vi "Engine-Throttle-Host.vi"() -> ()   [LabVIEW 2016]
panel:
  in  "_Hidden":enum32{"Page 1"}(tab)
  out "TB1_DisHHChans":sgl[](array[numeric])
  out "TB2_DisHHChans":sgl[](array[numeric])
  out "TB1_DC":sgl
  out "TB2_DC":sgl
  out "TB1_Polarity":bool
  out "TB2_Polarity":bool
  out "TB1_Fault":bool
  out "TB2_Fault":bool
  out "TB2_ModeStatus":T1(ring)
  in  "TB2_ModeSelect":T1(ring)
  in  "TB2_ControlEnable":bool
  in  "TB2_Psn_Req":sgl caption="TB1_PsnReq" format="%3_3g"
  out "TB2_Primary":sgl format="%3_3g"
  in  "TB1_ModeSelect":T1(ring)
  out "TB1_Primary":sgl format="%3_3g"
  in  "TB1_ControlEnable":bool
  in  "TB1_Psn_Req":sgl caption="TB1_PsnReq" format="%3_3g"
  out "TB1_ModeStatus":T1(ring)
  in  "_ThrottleTab":enum32{"Throttle 1", "Throttle 2"}(tab)
  in  "_ParameterTab":T2(tab)
  in  "TB1_CtrlCal":T3={"TLead [sec]"=0.0, "TLag [sec]"=0.1, "KRpos [V/ ]"=0.5, "TIpos [sec]"=0.15, "TDpos [sec]"=0.01, "KRneg [V/ ]"=1.0, "TIneg [sec]"=0.1, "TDneg [sec]"=0.001, "LH Position Band"=0.2, "U LH (V)"=2.0, "U LH Lag [sec]"=0.06, "US (V)"=0.5, "US Lag [sec]"=0.15, "LH Position"=5.0, "Motor Resistance"=2.4, "Position Fault Thresh"=10.0} caption="Control Calibration" {"LH Position" format="%.3f"; "U LH Lag [sec]" format="%.3f"; "US Lag [sec]" format="%.3f"; "TLead [sec]" format="%.3f"; "TLag [sec]" format="%.3f"}
  in  "TB1_PsnCalIn":T4 caption="Position Calibration In"
  in  "TB1_PsnCalSettings":T5={"Psn Cal Init Delay (sec)"=1.0, "u Psn Cal Inc (V)"=0.2, "u Psn Cal Inc Thresh (V)"=1.1, "Psn Cal Return From Pos Delay (sec)"=1.0, "u Psn Cal Dec Thresh (V)"=-1.1, "u Psn Cal Dec (V)"=-0.2, "Psn Cal Return From Neg Delay (sec)"=1.0, "u Psn Cal Pos Init (V)"=3.4, "u Psn Cal Neg Init (V)"=-3.0, "Psn Cal Offset (V)"=0.015, "Psn Cal Diff Thresh (V)"=3.0} caption="Position Calibration Settings" {"Psn Cal Diff Thresh (V)" min=0; "Psn Cal Offset (V)" min=0; "u Psn Cal Neg Init (V)" max=0; "u Psn Cal Pos Init (V)" min=0; "Psn Cal Return From Neg Delay (sec)" min=0; "u Psn Cal Dec (V)" max=0; "u Psn Cal Dec Thresh (V)" max=0; "Psn Cal Return From Pos Delay (sec)" min=0; "u Psn Cal Inc Thresh (V)" min=0; "u Psn Cal Inc (V)" min=0; "Psn Cal Init Delay (sec)" min=0}
  in  "TB1_Init":bool
  out "TB1_PsnCalOut":T6={"Primary Analog Range (V)"=[], "Secondary Analog Range (V)"=[], "Position Range"=[], "Position Calibrated"=FALSE, "Pos Cal Return From Positive Delay (sec)"=0.1, "Pos Cal Init Delay (sec)"=0.0, "u Limit Positive"=FALSE, "u Limit Negative"=FALSE, "Pos Cal Diff Fault"=FALSE} caption="Position Calibration Out" {"Pos Cal Init Delay (sec)" format="%.3f"; "Pos Cal Return From Positive Delay (sec)" format="%.3f"}
  in  "TB1_PWMFreq":sgl caption="[Hz]"
  in  "TB1_FullHChanSelect":i32(ring) caption="Output Channels" items=["None"=-2, "HH 1+HH 2"=0, "HH 2+HH 3"=1, "HH 3+HH 4"=2, "HH 4+HH 5"=3, "HH 5+HH 6"=4, "HH 6+HH 7"=5, "HH 7+HH 8"=6, "HH 8+HH 9"=7, "HH 9+HH 10"=8, "HH 10+HH 11"=9, "HH 11+HH 12"=10]
  out "TB1_Analog2":sgl caption="Analog 2 Select"
  out "TB1_Analog1":sgl caption="Analog 1 Select"
  in  "TB1_Analog2Index":i32(ring) caption="Analog 2 Select" items=["None"=-1, "AI 1"=0, "AI 2"=1, "AI 3"=2, "AI 4"=3, "AI 5"=4, "AI 6"=5, "AI 7"=6, "AI 8"=7, "AI 9"=8, "AI 10"=9, "AI 11"=10, "AI 12"=11]
  in  "TB1_Analog1Index":i32(ring) caption="Analog 1 Select" items=["AI 1", "AI 2", "AI 3", "AI 4", "AI 5", "AI 6", "AI 7", "AI 8", "AI 9", "AI 10", "AI 11", "AI 12"]
  in  "TB1_PrimarySelect":bool caption="Primary Select"
  out "TB1_Analog2Unit":string
  out "TB1_Analog1Unit":string
  out "TB1_CtrlData":T7 caption="Throttle Status" {"uLHc (V)" format="%.2f"; "uFc (V)" format="%.2f"; "uPID (V)" format="%.2f"}
  in  "_ParameterTab2":T2(tab)
  in  "TB2_CtrlCal":T3={"TLead [sec]"=0.0, "TLag [sec]"=0.1, "KRpos [V/ ]"=0.5, "TIpos [sec]"=0.15, "TDpos [sec]"=0.01, "KRneg [V/ ]"=1.0, "TIneg [sec]"=0.1, "TDneg [sec]"=0.001, "LH Position Band"=0.2, "U LH (V)"=2.0, "U LH Lag [sec]"=0.06, "US (V)"=0.5, "US Lag [sec]"=0.15, "LH Position"=5.0, "Motor Resistance"=2.4, "Position Fault Thresh"=10.0} caption="Control Calibration" {"LH Position" format="%.3f"; "U LH Lag [sec]" format="%.3f"; "US Lag [sec]" format="%.3f"; "TLead [sec]" format="%.3f"; "TLag [sec]" format="%.3f"}
  in  "TB2_PsnCalSettings":T5={"Psn Cal Init Delay (sec)"=1.0, "u Psn Cal Inc (V)"=0.2, "u Psn Cal Inc Thresh (V)"=1.1, "Psn Cal Return From Pos Delay (sec)"=1.0, "u Psn Cal Dec Thresh (V)"=-1.1, "u Psn Cal Dec (V)"=-0.2, "Psn Cal Return From Neg Delay (sec)"=1.0, "u Psn Cal Pos Init (V)"=3.4, "u Psn Cal Neg Init (V)"=-3.0, "Psn Cal Offset (V)"=0.015, "Psn Cal Diff Thresh (V)"=3.0} caption="Position Calibration Settings" {"Psn Cal Diff Thresh (V)" min=0; "Psn Cal Offset (V)" min=0; "u Psn Cal Neg Init (V)" max=0; "u Psn Cal Pos Init (V)" min=0; "Psn Cal Return From Neg Delay (sec)" min=0; "u Psn Cal Dec (V)" max=0; "u Psn Cal Dec Thresh (V)" max=0; "Psn Cal Return From Pos Delay (sec)" min=0; "u Psn Cal Inc Thresh (V)" min=0; "u Psn Cal Inc (V)" min=0; "Psn Cal Init Delay (sec)" min=0}
  in  "TB2_PsnCalIn":T4 caption="Position Calibration In"
  in  "TB2_Init":bool
  out "TB2_PsnCalOut":T6={"Primary Analog Range (V)"=[], "Secondary Analog Range (V)"=[], "Position Range"=[], "Position Calibrated"=FALSE, "Pos Cal Return From Positive Delay (sec)"=0.1, "Pos Cal Init Delay (sec)"=0.0, "u Limit Positive"=FALSE, "u Limit Negative"=FALSE, "Pos Cal Diff Fault"=FALSE} caption="Position Calibration Out" {"Pos Cal Init Delay (sec)" format="%.3f"; "Pos Cal Return From Positive Delay (sec)" format="%.3f"}
  in  "TB2_PWMFreq":sgl caption="[Hz]"
  in  "TB2_FullHChanSelect":i32(ring) caption="Output Channels" items=["None"=-2, "HH 1+HH 2"=0, "HH 2+HH 3"=1, "HH 3+HH 4"=2, "HH 4+HH 5"=3, "HH 5+HH 6"=4, "HH 6+HH 7"=5, "HH 7+HH 8"=6, "HH 8+HH 9"=7, "HH 9+HH 10"=8, "HH 10+HH 11"=9, "HH 11+HH 12"=10]
  out "TB2_Analog2":sgl caption="Analog 2 Select"
  out "TB2_Analog1":sgl caption="Analog 1 Select"
  in  "TB2_Analog2Index":i32(ring) caption="Analog 2 Select" items=["None"=-1, "AI 1"=0, "AI 2"=1, "AI 3"=2, "AI 4"=3, "AI 5"=4, "AI 6"=5, "AI 7"=6, "AI 8"=7, "AI 9"=8, "AI 10"=9, "AI 11"=10, "AI 12"=11]
  in  "TB2_Analog1Index":i32(ring) caption="Analog 1 Select" items=["AI 1", "AI 2", "AI 3", "AI 4", "AI 5", "AI 6", "AI 7", "AI 8", "AI 9", "AI 10", "AI 11", "AI 12"]
  in  "TB2_PrimarySelect":bool caption="Primary Select"
  out "TB2_Analog1Unit":string
  out "TB2_Analog2Unit":string
  out "TB2_CtrlData":T7 caption="Throttle Status" {"uLHc (V)" format="%.2f"; "uFc (V)" format="%.2f"; "uPID (V)" format="%.2f"}
  in  "_SettingsSelect":i32(listbox)
  in  "_AdvancedSettings":bool caption="Advanced Settings"
  in  "_ThrottleData":i32(listbox)
  # "Electronic Throttle Body Control"
  # "Throttle 2 Control"
  # "Enable"
  # "Request"
  # "Primary"
  # "Mode"
  # "Throttle 1 Control"
  # "Enable"
  # "Request"
  # "Primary"
  # "Mode"
  # "Input Channels Setup"
  # "Output Channels Setup"
  # "PWM Frequency"
  # "Input Channels Setup"
  # "Output Channels Setup"
  # "PWM Frequency"
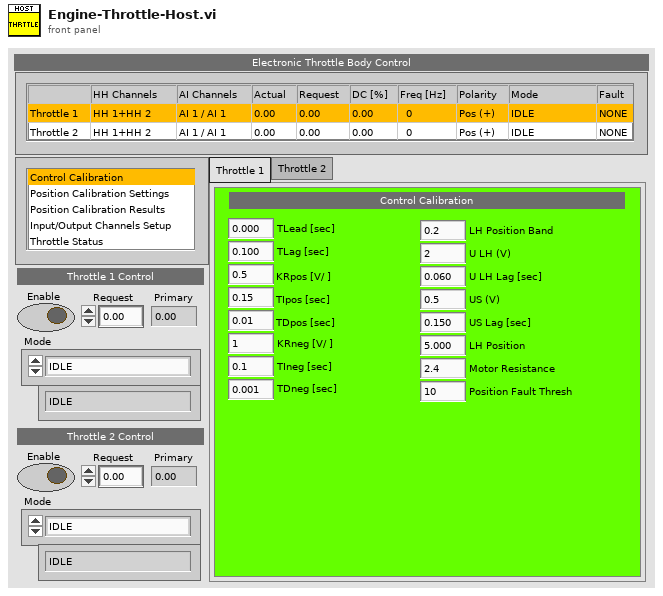
[diagram p1: front panel]
types:
  T1 = enum16{"IDLE", "POSITION CALIBRATION", "CONTROL CALIBRATION", "CONTROL"}
  T2 = enum32{"Control", "Psn Cal Settings", "Psn Cal Results", "Input / Output", "Status"}
  T3 = cluster{"TLead [sec]":sgl, "TLag [sec]":sgl, "KRpos [V/ ]":sgl, "TIpos [sec]":sgl, "TDpos [sec]":sgl, "KRneg [V/ ]":sgl, "TIneg [sec]":sgl, "TDneg [sec]":sgl, "LH Position Band":sgl, "U LH (V)":sgl, "U LH Lag [sec]":sgl, "US (V)":sgl, "US Lag [sec]":sgl, "LH Position":sgl, "Motor Resistance":sgl, "Position Fault Thresh":sgl}
  T4 = cluster{"Analog1 [V]":sgl[], "Analog2 [V]":sgl[], "Position":sgl[]}
  T5 = cluster{"Psn Cal Init Delay (sec)":sgl, "u Psn Cal Inc (V)":sgl, "u Psn Cal Inc Thresh (V)":sgl, "Psn Cal Return From Pos Delay (sec)":sgl, "u Psn Cal Dec Thresh (V)":sgl, "u Psn Cal Dec (V)":sgl, "Psn Cal Return From Neg Delay (sec)":sgl, "u Psn Cal Pos Init (V)":sgl, "u Psn Cal Neg Init (V)":sgl, "Psn Cal Offset (V)":sgl, "Psn Cal Diff Thresh (V)":sgl}
  T6 = cluster{"Primary Analog Range (V)":sgl[], "Secondary Analog Range (V)":sgl[], "Position Range":sgl[], "Position Calibrated":bool, "Pos Cal Return From Positive Delay (sec)":sgl, "Pos Cal Init Delay (sec)":sgl, "u Limit Positive":bool, "u Limit Negative":bool, "Pos Cal Diff Fault":bool}
  T7 = cluster{"Primary Position":sgl, "Secondary Position":sgl, "AboveLH?":bool, "Position Fault":bool, "u Limit?":bool, "uLHc (V)":sgl, "uFc (V)":sgl, "uPID (V)":sgl, "u (V)":sgl}
  T8 = enum8{"Enabled", "Disabled", "Disabled and Grayed Out"}
  T9 = cluster{"HH":string, "Primary":string, "Second":string, "PriPsn":sgl, "ReqPsn":sgl, "DC":sgl, "Freq":sgl, "Polarity":bool, "Mode":enum16{"IDLE", "POSITION CALIBRATION", "CONTROL CALIBRATION", "CONTROL"}, "Fault":bool}
  T10 = cluster{"HH":string, "Primary":string, "Second":string, "PriPsn":sgl, "ReqPsn":sgl, "DC":sgl, "Freq":sgl, "Polarity":bool, "Mode":enum16{"IDLE", "POSITION CALIBRATION", "CONTROL CALIBRATION", "CONTROL"}, "Fault":bool}[]
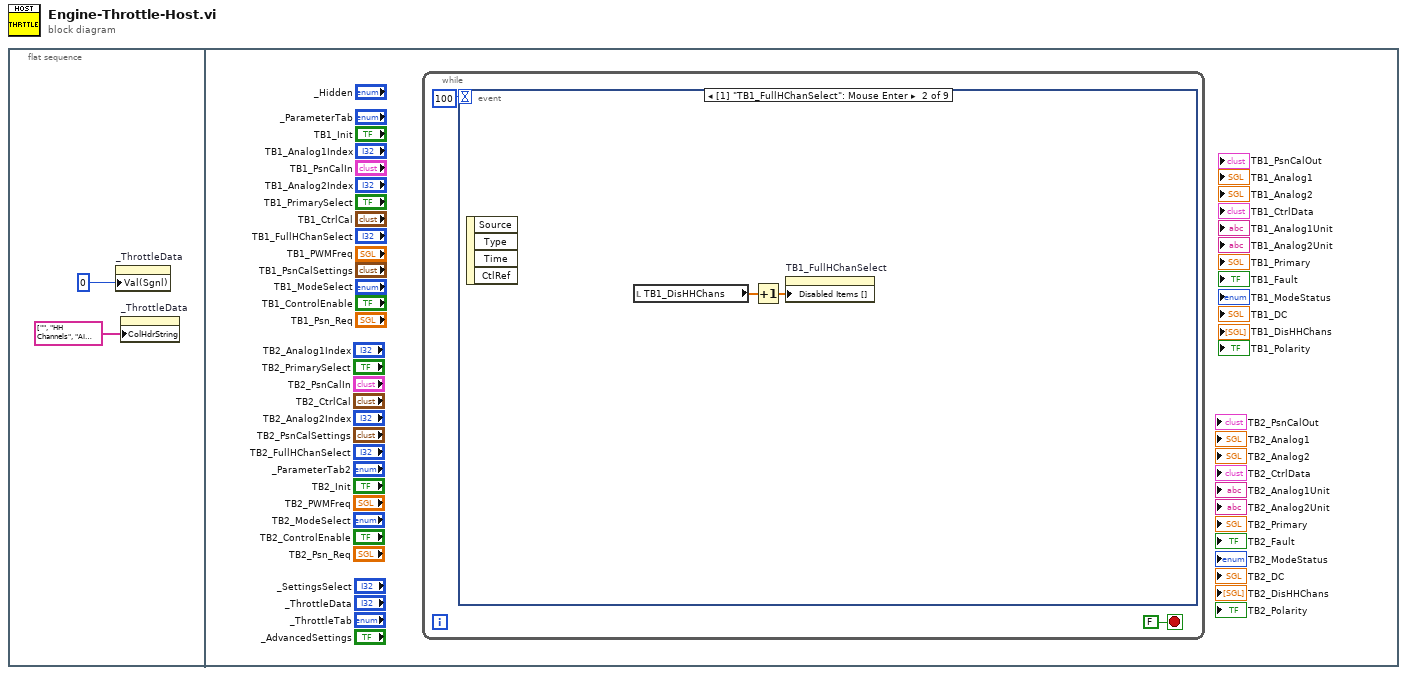
[diagram p0: block diagram]
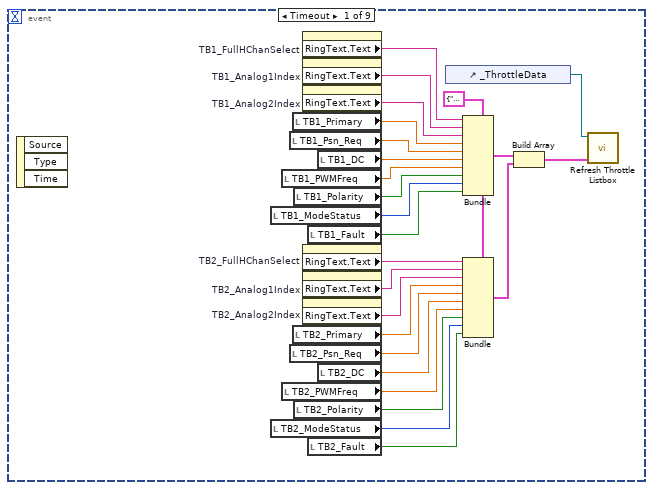
[diagram p2: hidden frame]
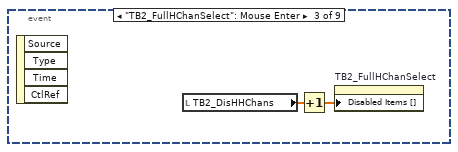
[diagram p3: hidden frame]
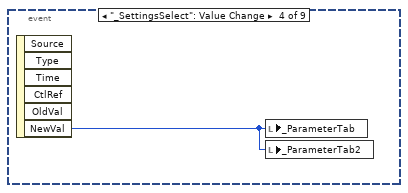
[diagram p4: hidden frame]
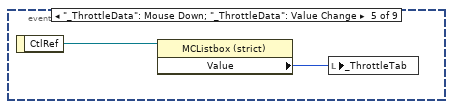
[diagram p5: hidden frame]
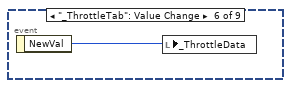
[diagram p6: hidden frame]
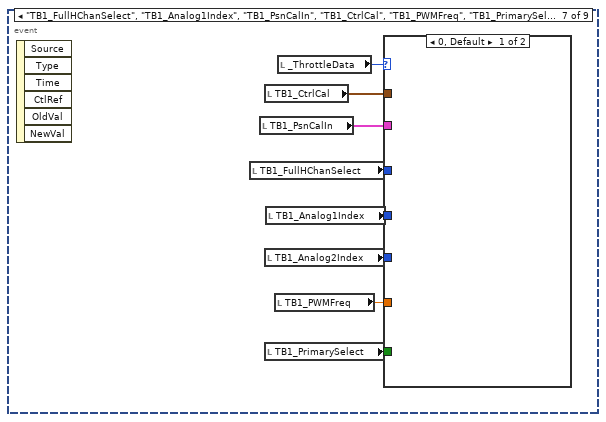
[diagram p7: hidden frame]
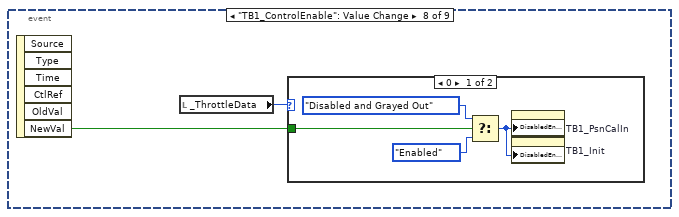
[diagram p9: hidden frame]
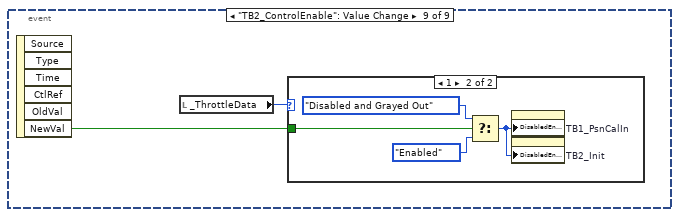
[diagram p11: hidden frame]
diagram:
  n1 = flat-sequence {
    frame #0 {
      n2 = property on="_ThrottleData" class="MCListbox (strict)"("Val(Sgnl)"=0 ("_Throttle Data")) -> ()  [unwired: 2 in, 2 out]
      n3 = property on="_ThrottleData" class="MCListbox (strict)"("ColHdrString"=string[] ["", "HH Channels", "AI Channels", "Actual", "Request", "DC [%]", "Freq [Hz]", "Polarity", "Mode", "Fault"] ("Row Header Strings[]")) -> ()  [unwired: 2 in, 2 out]
    }
    frame #1 {
      n4 = while {
        stop <- FALSE stop-if-true
        n5 = event shown="[1] \"TB1_FullHChanSelect\": Mouse Enter" {
          selector: _ -> [_ _ _ _ _ _ _ _ _]
          dyn-events: _ -> [_ _ _ _ _ _ _ _ _]
          timeout: 100 -> [_ _ _ _ _ _ _ _ _]
          event Timeout {
            w9 = T9 {"HH"="", "Primary"="", "Second"="", "PriPsn"=0.0, "ReqPsn"=0.0, "DC"=0.0, "Freq"=0.0, "Polarity"=FALSE, "Mode"=enum."IDLE", "Fault"=FALSE} ("Data")
            n6 = event-data() -> ()  [unwired: 1 in, 3 out]
            n7 = local read "TB1_ModeStatus"() -> (w8:T1)
            n8 = local read "TB2_ModeStatus"() -> (w7:T1)
            n9 = local read "TB1_PWMFreq"() -> (w17:sgl)
            n10 = local read "TB2_PWMFreq"() -> (w16:sgl)
            n11 = local read "TB1_Psn_Req"() -> (w25:sgl)
            n12 = local read "TB2_Psn_Req"() -> (w20:sgl)
            n13 = local read "TB1_Primary"() -> (w26:sgl)
            n14 = local read "TB2_Primary"() -> (w19:sgl)
            n15 = local read "TB1_Polarity"() -> (w23:bool)
            n16 = local read "TB2_Polarity"() -> (w22:bool)
            n17 = property on="TB1_FullHChanSelect" class="Ring (strict)"() -> ("RingText.Text"=w10:string)  [unwired: 2 in, 2 out]
            n18 = property on="TB1_Analog1Index" class="Ring (strict)"() -> ("RingText.Text"=w11:string)  [unwired: 2 in, 2 out]
            n19 = property on="TB1_Analog2Index" class="Ring (strict)"() -> ("RingText.Text"=w12:string)  [unwired: 2 in, 2 out]
            n20 = property on="TB2_FullHChanSelect" class="Ring (strict)"() -> ("RingText.Text"=w13:string)  [unwired: 2 in, 2 out]
            n21 = property on="TB2_Analog1Index" class="Ring (strict)"() -> ("RingText.Text"=w14:string)  [unwired: 2 in, 2 out]
            n22 = property on="TB2_Analog2Index" class="Ring (strict)"() -> ("RingText.Text"=w15:string)  [unwired: 2 in, 2 out]
            n23 = local read "TB1_Fault"() -> (w6:bool)
            n24 = local read "TB2_Fault"() -> (w5:bool)
            n25 = local read "TB1_DC"() -> (w24:sgl)
            n26 = local read "TB2_DC"() -> (w21:sgl)
            n27 = control-ref of="_ThrottleData"() -> (w29:refnum<vi>)
            n28 = Bundle(cluster=w9, "HH"=w10, "Primary"=w11, "Second"=w12, "PriPsn"=w26, "ReqPsn"=w25, "DC"=w24, "Freq"=w17, "Polarity"=w23, "Mode"=w8, "Fault"=w6) -> (w28:T9)
            n29 = Bundle(cluster=w9, "HH"=w13, "Primary"=w14, "Second"=w15, "PriPsn"=w19, "ReqPsn"=w20, "DC"=w21, "Freq"=w16, "Polarity"=w22, "Mode"=w7, "Fault"=w5) -> (w27:T9)
            n30 = Build Array(w28, w27) -> (w18:T10)
            n31 = call "Refresh Throttle Listbox.vi"("Data"=w18, "Throttle Data"=w29) -> ()  [unwired: 10 in]
          }
          event "TB1_FullHChanSelect": Mouse Enter {
            n32 = event-data() -> ()  [unwired: 1 in, 4 out]
            n33 = local read "TB1_DisHHChans"() -> (w31:sgl[])
            n34 = Increment(x=w31) -> (x+1=w30:sgl[])
            n35 = property on="TB1_FullHChanSelect" class="Ring (strict)"("Disabled Items []"=w30) -> ()  [unwired: 2 in, 2 out]
          }
          event "TB2_FullHChanSelect": Mouse Enter {
            n36 = event-data() -> ()  [unwired: 1 in, 4 out]
            n37 = local read "TB2_DisHHChans"() -> (w33:sgl[])
            n38 = Increment(x=w33) -> (x+1=w32:sgl[])
            n39 = property on="TB2_FullHChanSelect" class="Ring (strict)"("Disabled Items []"=w32) -> ()  [unwired: 2 in, 2 out]
          }
          event "_SettingsSelect": Value Change {
            n40 = event-data() -> ("NewVal"=w34:i32)  [unwired: 1 in, 5 out]
            n41 = local write "_ParameterTab"(w34) -> ()
            n42 = local write "_ParameterTab2"(w34) -> ()
          }
          event "_ThrottleData": Mouse Down; "_ThrottleData": Value Change {
            n43 = event-data() -> ("CtlRef"=w36:refnum<vi>)  [unwired: 1 in]
            n44 = property class="MCListbox (strict)"(reference=w36) -> ("Value"=w35:i32)  [unwired: 1 in, 2 out]
            n45 = local write "_ThrottleTab"(w35) -> ()
          }
          event "_ThrottleTab": Value Change {
            n46 = event-data() -> ("NewVal"=w37:enum32{"Throttle 1", "Throttle 2"})  [unwired: 1 in]
            n47 = local write "_ThrottleData"(w37) -> ()
          }
          event "TB1_FullHChanSelect", "TB1_Analog1Index", "TB1_PsnCalIn", "TB1_CtrlCal", "TB1_PWMFreq", "TB1_PrimarySelect", "TB1_Analog2Index": Value Change {
            n48 = event-data() -> ()  [unwired: 1 in, 6 out]
            n49 = local read "TB1_FullHChanSelect"() -> (w43:i32)
            n50 = local read "TB1_PsnCalIn"() -> (w41:T4)
            n51 = local read "TB1_CtrlCal"() -> (w44:T3)
            n52 = local read "TB1_Analog2Index"() -> (w40:i32)
            n53 = local read "TB1_PrimarySelect"() -> (w38:bool)
            n54 = local read "TB1_Analog1Index"() -> (w42:i32)
            n55 = local read "TB1_PWMFreq"() -> (w39:sgl)
            n56 = local read "_ThrottleData"() -> (w45:i32)
            n57 = case shown="0, Default" w45 {
              tunnel: w44 -> [_ _]
              tunnel: w43 -> [_ _]
              tunnel: w42 -> [_ _]
              tunnel: w41 -> [_ _]
              tunnel: w40 -> [_ _]
              tunnel: w39 -> [_ _]
              tunnel: w38 -> [_ _]
              frame 0, Default {
              }
              frame 1 {
              }
            }
          }
          event "TB1_ControlEnable": Value Change {
            n58 = event-data() -> ("NewVal"=w46:bool)  [unwired: 1 in, 5 out]
            n59 = local read "_ThrottleData"() -> (w47:i32)
            n60 = case shown="0" w47 {
              tunnel: w46 -> [w49 _]
              frame 0 {
                n61 = Select(t=T8."Disabled and Grayed Out" ("Disabled"), s=w49, f=T8."Enabled" ("Disabled")) -> (s? t:f=w48:T8)
                n62 = property on="TB1_PsnCalIn" class="Clust (strict)"("DisabledEnum"=w48) -> ()  [unwired: 2 in, 2 out]
                n63 = property on="TB1_Init" class="Bool (strict)"("DisabledEnum"=w48) -> ()  [unwired: 2 in, 2 out]
              }
              frame 1, Default {
              }
            }
          }
          event "TB2_ControlEnable": Value Change {
            n64 = event-data() -> ("NewVal"=w52:bool)  [unwired: 1 in, 5 out]
            n65 = local read "_ThrottleData"() -> (w53:i32)
            n66 = case shown="1" w53 {
              tunnel: w52 -> [_ w55]
              frame 0, Default {
              }
              frame 1 {
                n67 = Select(t=T8."Disabled and Grayed Out" ("Disabled"), s=w55, f=T8."Enabled" ("Disabled")) -> (s? t:f=w54:T8)
                n68 = property on="TB1_PsnCalIn" class="Clust (strict)"("DisabledEnum"=w54) -> ()  [unwired: 2 in, 2 out]
                n69 = property on="TB2_Init" class="Bool (strict)"("DisabledEnum"=w54) -> ()  [unwired: 2 in, 2 out]
              }
            }
          }
        }
      }
    }
  }
